vi "LoadWaveString.vi"(0 "Wave String":string, 1 "Wave (MHz,us,Pi)":string[][](array[string])) -> (2 "All Wave (MHz,us)":string[][](table)=[["Frequency (MHz)", "Duration (us)", "Amplitude", "Phase (Pi)", "Gap (us)"], ["200.012", "100.000", "1.000", "0.000", "0.001"]], 3 "All Wave":T1 {"Phase (Pi)" min=-1.0 max=1.0 step=0.1 format="%.2f"; "Gap (us)" format="%.2f"; "Amplitude" format="%.2f"; "Duration (us)" format="%.2f"; "Frequency (MHz)" format="%.4f"}, 4 "SegmentPositions":i32[](array[numeric]))   [LabVIEW 2014]
uses:
  Wave.ctl
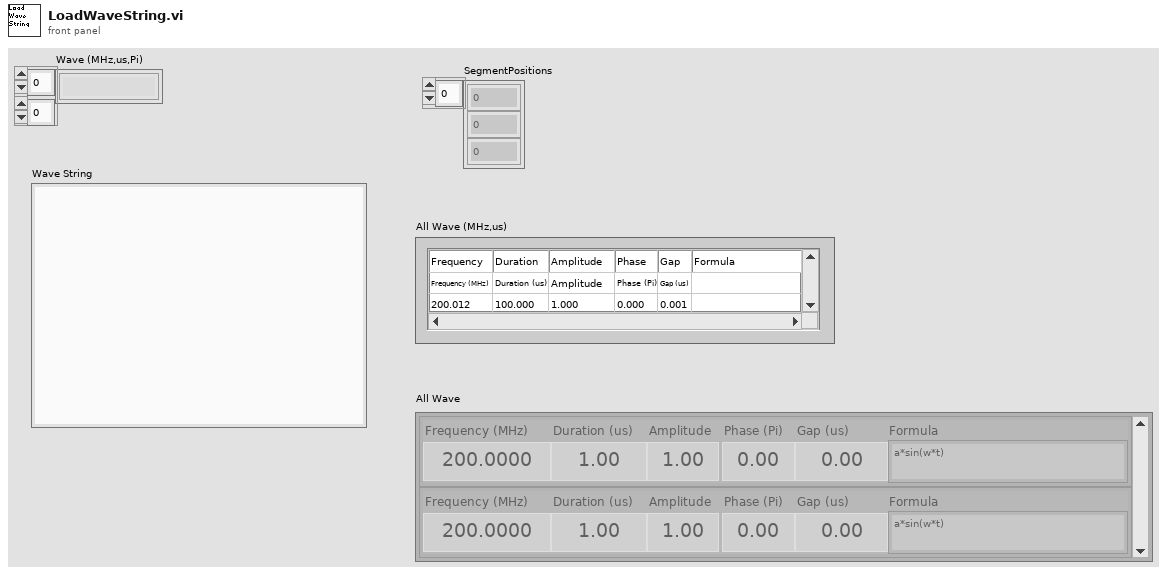
[diagram p1: front panel]
types:
  T1 = typedef "Wave.ctl" = cluster{"Frequency (MHz)":dbl, "Duration (us)":dbl, "Amplitude":dbl, "Phase (Pi)":dbl, "Gap (us)":dbl, "Formula":string}[]
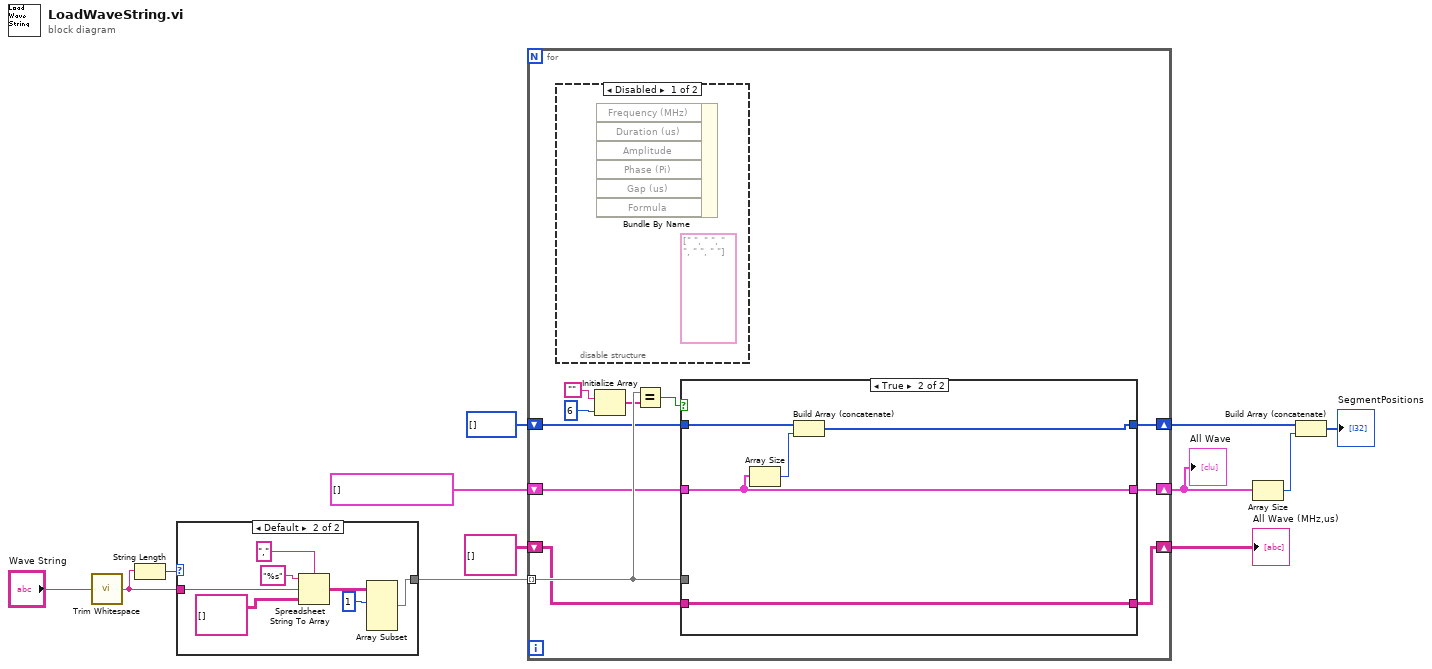
[diagram p0: block diagram]
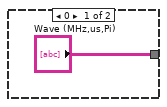
[diagram p2: hidden frame]
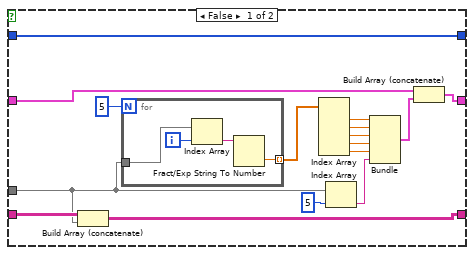
[diagram p4: hidden frame]
diagram:
  n1 = call <vilib>:"Trim Whitespace.vi"("string"="Wave String") -> ("trimmed string"=w2:string)  [unwired: 1 in]
  n2 = String Length(string=w2) -> (length=w1:i32)
  n3 = case shown="Default" w1 {
    tunnel: ["Wave (MHz,us,Pi)" w15] -> w4
    tunnel: w2 -> [_ w14]
    frame 0 {
    }
    frame Default {
      n4 = Spreadsheet String To Array(delimiter (Tab)="," ("delimiter (\\t)"), format string="%s", spreadsheet string=w14, array type (2D Dbl)=string[][] [] ("Wave (MHz, us, Pi)")) -> (array=w17:string[][])
      n5 = Array Subset(array=w17, index (row)=1 ("index")) -> (w15:string[][])  [unwired: 3 in]
    }
  }
  n6 = for {
    tunnel: w4 -> [w31] mode=indexing
    shift-right: [w26] -> w7
    shift-left: string[][] [] ("All Wave (MHz,us)") -> [w27]
    shift-right: [w24] -> w11
    shift-left: i32[] [] ("appended array") -> [w25]
    shift-right: [w21] -> w5
    shift-left: T1 [] ("All Wave") -> [w22]
    n7 = disable-structure shown="Disabled" {
      frame Disabled {
        (unwired) string[] [" ", " ", " ", " ", " "] ("y")
        n8 = Bundle By Name() -> ()  [unwired: 7 in, 1 out]
      }
      frame Enabled {
      }
    }
    n9 = Initialize Array("", 6 ("dimension size")) -> (w28:string[])
    n10 = Equal?(x=w31, y=w28) -> (x = y?=w23:bool)
    n11 = case shown="True" w23 {
      tunnel: w31 -> [w40 _]
      tunnel: [w47 w56] -> w26
      tunnel: w27 -> [w46 w56]
      tunnel: w25 -> [w45 w55]
      tunnel: [w45 w53] -> w24
      tunnel: w22 -> [w43 w52]
      tunnel: [w42 w52] -> w21
      frame False {
        n12 = Build Array (concatenate)(w46, w40) -> (w47:string[][])
        n13 = for {
          N: 5 -> [_]
          tunnel: [w51] -> w41 mode=indexing
          tunnel: w40 -> [w50]
          i -> [w49]
          n14 = Index Array(array=w50, index=w49) -> (element=w48:string)
          n15 = Fract/Exp String To Number(string=w48) -> (number=w51:dbl)  [unwired: 3 in, 1 out]
        }
        n16 = Index Array(array=w41) -> (element #1=w38:dbl, element #2=w37:dbl, element #3=w36:dbl, element #4=w35:dbl, element #5=w34:dbl)  [unwired: 5 in]
        n17 = Index Array(array=w40, index=5) -> (element=w33:string)
        n18 = Bundle(w38, w37, w36, w35, w34, w33) -> (w32:cluster{dbl, dbl, dbl, dbl, dbl, string})  [unwired: 1 in]
        n19 = Build Array (concatenate)(w43, w32) -> (w42:T1)
      }
      frame True {
        n20 = Array Size(array=w52) -> (size(s)=w54:i32)
        n21 = Build Array (concatenate)(w55, w54) -> (w53:i32[])
      }
    }
  }
  "All Wave (MHz,us)" <- w7
  "All Wave" <- w5
  n22 = Array Size(array=w5) -> (size(s)=w10:i32)
  n23 = Build Array (concatenate)(w11, w10) -> (→"SegmentPositions":i32[])
